vi "Destroy Message Transport.vi"(8 "error in":errorcluster, 11 "QueueMessageTransport in":refnum<class "QueueMessageTransport.lvclass">) -> (0 "error out":errorcluster, 3 "QueueMessageTransport out":refnum<class "QueueMessageTransport.lvclass">)   [LabVIEW 2016, in "QueueMessageTransport.lvclass"]
uses:
  QueueMessageTransport.lvclass
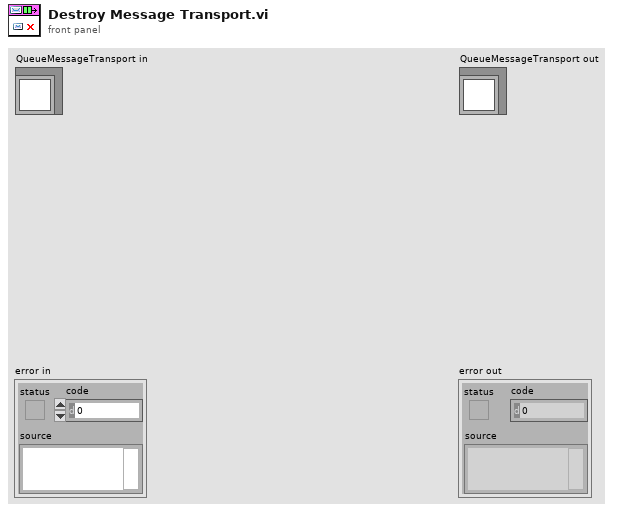
[diagram p1: front panel]
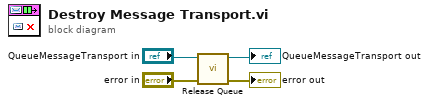
[diagram p0: block diagram]
diagram:
  n1 = call "Release Queue.vi"("error in"="error in", "QueueMessageTransport in"="QueueMessageTransport in") -> ("error out"=→"error out":errorcluster, "QueueMessageTransport out"=→"QueueMessageTransport out":refnum<class "QueueMessageTransport.lvclass">)  [unwired: 8 in]
